vi "StartMeas.vi"(8 "error in (no error)":errorcluster, 11 "PacificPowerSource in":refnum<class "PacificPowerSource.lvclass">) -> (0 "error out":errorcluster, 3 "PacificPowerSource out":refnum<class "PacificPowerSource.lvclass">)   [LabVIEW 2018, in "AcPwrPlugins.lvlib" / "PacificPowerSource.lvclass"]
doc: "This VI starts the instrument measurement."
uses:
  PacificPowerSource.lvclass
  <instrlib>/Pacific Power UPC Series/Pacific Power UPC Series.lvlib
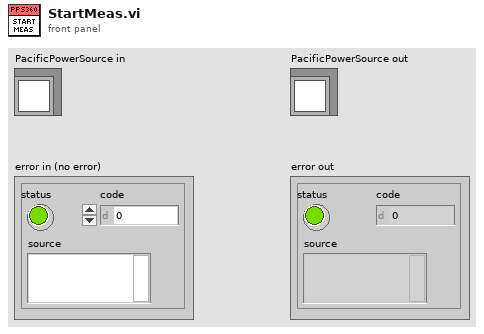
[diagram p1: front panel]
types:
  T1 = typedef "AcPwrPlugins.lvlib/PacificPowerSource.lvclass/LoadSettings.ctl" = cluster{"Handle":string, "Connected":bool, "Source Limits":cluster{"Frequency Minimum (45 Hz)":dbl, "Frequency Maximum (1200 Hz)":dbl, "Voltage Maximum (V)":dbl, "Voltage Minimum (V)":dbl, "Current Limit (40A)":dbl}, "Clear Device":bool, "Configure Output":cluster{"Coupling  (0: Direct)":u16, "Form (3: Three)":u16}, "Range Control (0: Auto)":u16, "Initial Voltage (0V)":u16, "Frequency":cluster{"Frequency Range (600Hz)":u16, "Frequency (45Hz)":dbl}, "Waveform":cluster{"Voltage Level (V)":dbl, "Phase (Degrees)":i32, "Channel Name (1: A)":u16, "Waveform (1: Sine)":u16}[], "Arbitrary Waveform":cluster{"Waveform Number (2: Arbitrary Waveform2)":u16, "Petcentage Of Voltages":dbl[]}, "Impedance Parameters (off, 0.00)":cluster{"State":bool, "Impedance":dbl}, "Waveform Type":bool, "Program Number":i32, "Transient Execution":bool}[]
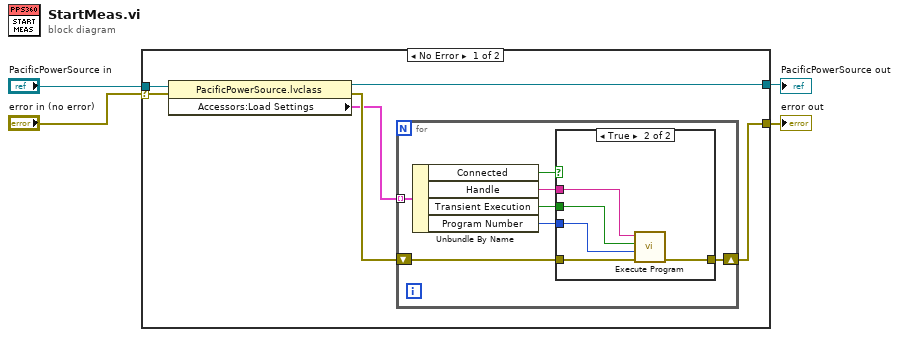
[diagram p0: block diagram]
diagram:
  n1 = case shown="No Error" "error in (no error)" {
    selector: "error in (no error)" -> [w9 w24]
    tunnel: "PacificPowerSource in" -> [w10 w25]
    tunnel: [w8 w25] -> w2
    tunnel: [w6 w24] -> w1
    frame No Error {
      n2 = property class="PacificPowerSource.lvclass"(reference=w10, error in=w9) -> (reference out=w8:refnum<class "PacificPowerSource.lvclass">, error out=w7:errorcluster, "Accessors:Load Settings"=w5:T1)
      n3 = for {
        shift-right: [w16] -> w6
        shift-left: w7 -> [w17]
        tunnel: w5 -> [w15] mode=indexing
        n4 = Unbundle By Name(w15) -> ("Connected"=w13:bool, "Handle"=w14:string, "Transient Execution"=w12:bool, "Program Number"=w11:i32)
        n5 = case shown="True" w13 {
          tunnel: w17 -> [w18 w23]
          tunnel: [w18 w22] -> w16
          tunnel: w14 -> [_ w21]
          tunnel: w12 -> [_ w20]
          tunnel: w11 -> [_ w19]
          frame False {
          }
          frame True {
            n6 = call <instrlib>:"Execute Program.vi"("error in (no error)"=w23, "Program Number (1)"=w19, "Enable Transient Execution (F: Disable)"=w20, "VISA resource name"=w21) -> ("error out"=w22:errorcluster)  [unwired: 6 in, 1 out]
          }
        }
      }
    }
    frame Error {
    }
  }
  "error out" <- w1
  "PacificPowerSource out" <- w2
